vi "sub_system_status.vi"(7 "Mode":enum16{"Initial", "Update", "Clear"}(ring)=enum."Update", 8 "error in":errorcluster, 9 "content":string, 10 "title":string, 11 "System Log":refnum<vi>) -> (0 "error out":errorcluster)   [LabVIEW 2018]
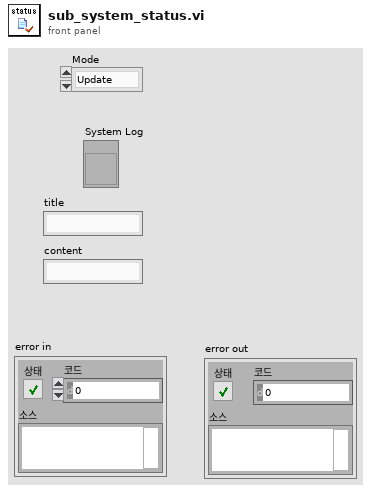
[diagram p1: front panel]
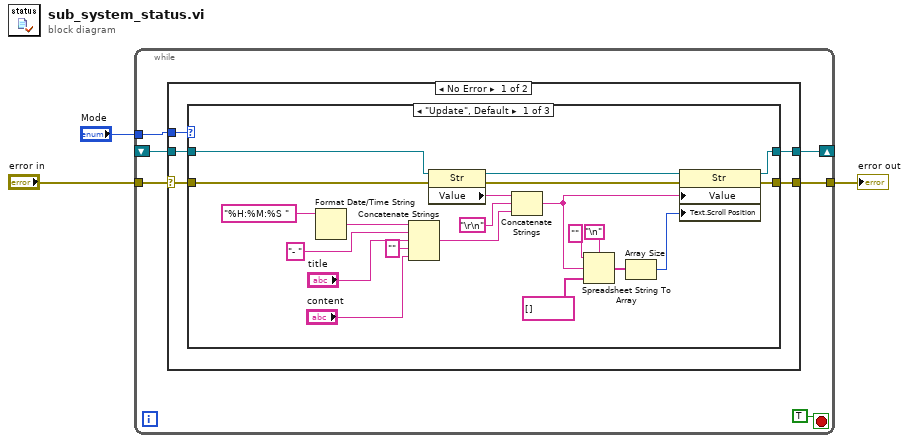
[diagram p0: block diagram]
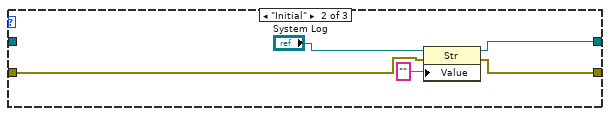
[diagram p2: hidden frame]
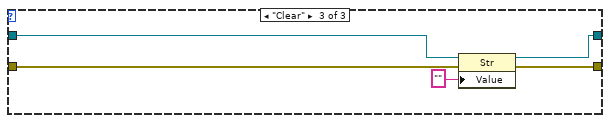
[diagram p3: hidden frame]
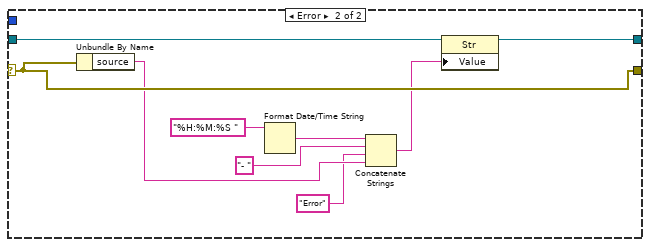
[diagram p4: hidden frame]
diagram:
  n1 = while {
    tunnel: "error in" -> [w4]
    tunnel: [w9] -> w2
    tunnel: "Mode" -> [w7]
    shift-right: [w6] -> _
    shift-left: _ -> [w5]
    stop <- TRUE stop-if-true
    n2 = case shown="No Error" w4 {
      selector: w4 -> [w10 w52]
      tunnel: [w14 w52] -> w9
      tunnel: w7 -> [w13 _]
      tunnel: [w12 w53] -> w6
      tunnel: w5 -> [w11 w54]
      frame No Error {
        n3 = case shown="\"Update\", Default" w13 {
          tunnel: w11 -> [w35 _ w43]
          tunnel: w10 -> [w30 w37 w45]
          tunnel: [w29 w38 w44] -> w14
          tunnel: [w28 w39 w42] -> w12
          frame "Update", Default {
            n4 = Format Date/Time String(time format string (%c)="%H:%M:%S " ("시간 포맷 문자열 (%c)")) -> (date/time string=w20:string)  [unwired: 2 in]
            n5 = Concatenate Strings(w20, "- " ("포맷 문자열"), "title", "" ("string"), "content") -> (w19:string)
            n6 = property class="Str"(reference=w35, error in=w30) -> (reference out=w32:refnum<vi>, error out=w31:errorcluster, "Value"=w34:string)
            n7 = Concatenate Strings(w34, "\r\n", w19) -> (w23:string)
            n8 = Spreadsheet String To Array(delimiter (Tab)="\n", format string="" ("포맷 문자열"), spreadsheet string=w23, array type (2D Dbl)=string[] []) -> (array=w27:string[])
            n9 = Array Size(array=w27) -> (size(s)=w22:i32)
            n10 = property class="Str"(reference=w32, error in=w31, "Value"=w23, "Text.Scroll Position"=w22) -> (reference out=w28:refnum<vi>, error out=w29:errorcluster)
          }
          frame "Initial" {
            n11 = property class="Str"(reference="System Log", error in=w37, "Value"="" ("값")) -> (reference out=w39:refnum<vi>, error out=w38:errorcluster)
          }
          frame "Clear" {
            n12 = property class="Str"(reference=w43, error in=w45, "Value"="" ("값")) -> (reference out=w42:refnum<vi>, error out=w44:errorcluster)
          }
        }
      }
      frame Error {
        n13 = Unbundle By Name(w52) -> ("source"=w47:string)
        n14 = Format Date/Time String(time format string (%c)="%H:%M:%S " ("시간 포맷 문자열 (%c)")) -> (date/time string=w50:string)  [unwired: 2 in]
        n15 = Concatenate Strings(w50, "- " ("포맷 문자열"), "Error" ("문자열"), w47) -> (w48:string)
        n16 = property class="Str"(reference=w54, "Value"=w48) -> (reference out=w53:refnum<vi>)  [unwired: 1 in, 1 out]
      }
    }
  }
  "error out" <- w2
